vi "Is There A Single Project Loaded In Memory.vi"(8 "Error In":errorcluster) -> (0 "Error Out":errorcluster, 2 "My Computer ProjectItem Ref":refnum<vi>, 3 "A Single Project Loaded In Memory?":bool)   [LabVIEW 2022 SP3]
doc: "This VI returns True if and only if there's a single LabVIEW Project (lvproj) loaded (opened) in the application instance.\n\nThe VI will return False if the user has two or more LabVIEW Projects open at the same time."
panel:
  # "Development\nControls or indicators that are useful for development or testing, but which are not outputs of the VI."
  # "Input\nInputs to the VI"
  # "Output\nOutputs of the VI"
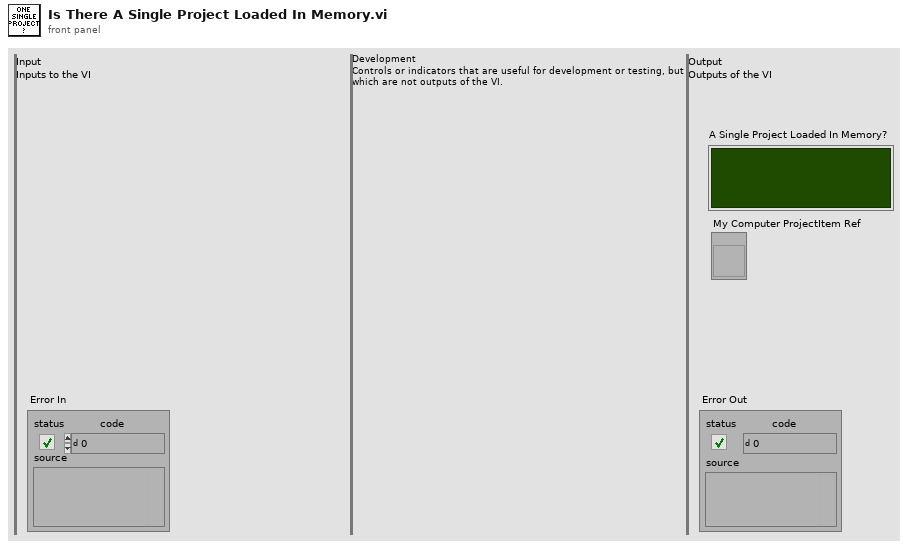
[diagram p1: front panel]
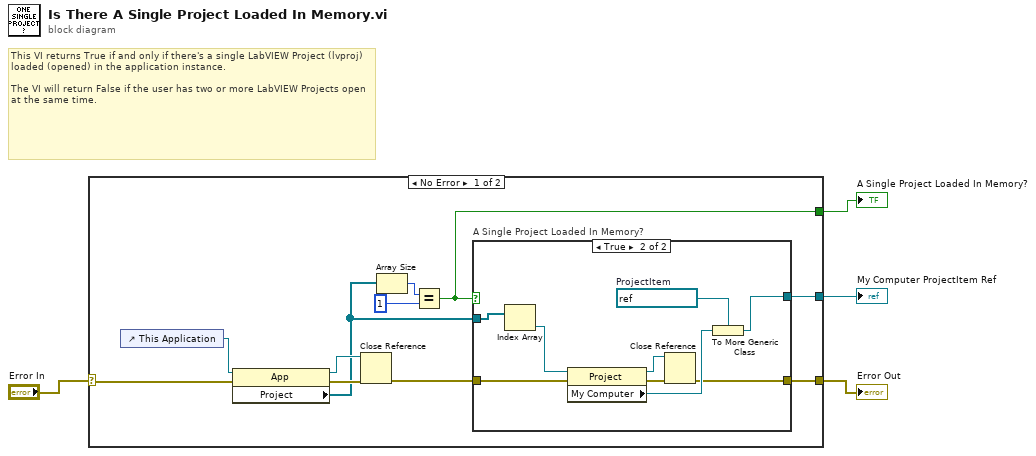
[diagram p0: block diagram]
diagram:
  # "This VI returns True if and only if there's a single LabVIEW Project (lvproj) loaded (opened) in the application instance.\n\nThe VI will return False if the user has two or more LabVIEW Projects open at the same time."
  n1 = case shown="No Error" "Error In" {
    selector: "Error In" -> [w12 w26]
    tunnel: [w8 w26] -> w3
    tunnel: [w7 _] -> w2
    tunnel: [w5 _] -> w1
    frame No Error {
      n2 = control-ref of="This Application"() -> (w14:refnum<vi>)
      n3 = property class="App"(reference=w14, error in=w12) -> (reference out=w13:refnum<vi>, error out=w15:errorcluster, "Project"=w6:refnum<vi>[])
      n4 = Close Reference(reference=w13, error in (no error)=w15) -> (error out=w11:errorcluster)
      n5 = Array Size(array=w6) -> (size(s)=w10:i32)
      n6 = Equal?(x=w10, y=1) -> (x = y?=w7:bool)
      n7 = case "A Single Project Loaded In Memory?" shown="True" w7 {
        tunnel: w11 -> [w16 w25]
        tunnel: [w16 w18] -> w8
        tunnel: w6 -> [_ w24]
        tunnel: [_ w19] -> w5
        frame False {
        }
        frame True {
          w20 = refnum<vi> refnum  # ProjectItem
          n8 = Index Array(array=w24) -> (element=w22:refnum<vi>)  [unwired: 1 in]
          n9 = property class="Project"(reference=w22, error in=w25) -> (reference out=w17:refnum<vi>, error out=w23:errorcluster, "My Computer"=w21:refnum<vi>)
          n10 = Close Reference(reference=w17, error in (no error)=w23) -> (error out=w18:errorcluster)
          n11 = To More Generic Class(target class=w20, reference=w21) -> (generic class reference=w19:refnum<vi>)
        }
      }
    }
    frame Error {
    }
  }
  "Error Out" <- w3
  "A Single Project Loaded In Memory?" <- w2
  "My Computer ProjectItem Ref" <- w1
